vi "CheckChecksum.vi"(8 "error in (no error)":errorcluster, 11 "CS++Message in":refnum<class "CS++Message.lvclass">) -> (0 "error out":errorcluster, 2 "ok?":bool, 3 "CS++Message out":refnum<class "CS++Message.lvclass">)   [LabVIEW 2015, in "CS++Message.lvlib" / "CS++Message.lvclass"]
uses:
  CS++Message.lvclass
  CS++Message.lvclass/CS++Message.ctl
  <vilib>/Utility/traverseref.llb/TRef TravTarget.ctl
  <vilib>/Utility/traverseref.llb/VI Scripting - Traverse.lvlib
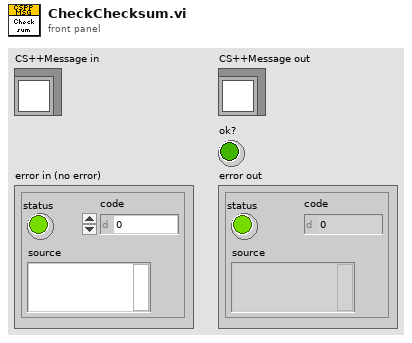
[diagram p1: front panel]
types:
  T1 = typedef "TRef TravTarget.ctl" = enum16{"FP", "BD", "Other"}
  T2 = typedef "imagedata.ctl" = cluster{"image type":i32, "image depth":i32, "image":u8[], "mask":u8[], "colors":u32[], "Rectangle":cluster{"left":i16, "top":i16, "right":i16, "bottom":i16}}
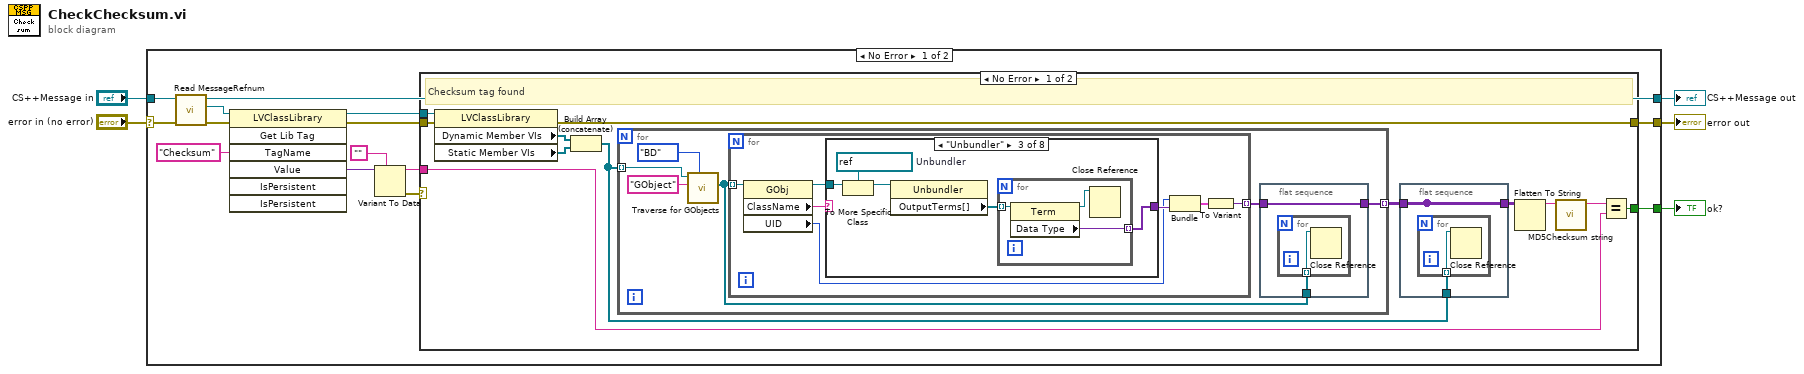
[diagram p0: block diagram]
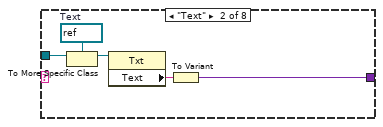
[diagram p3: hidden frame]
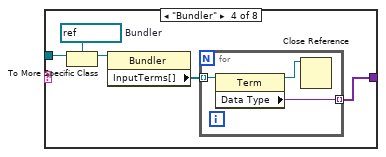
[diagram p4: hidden frame]
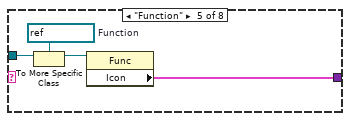
[diagram p5: hidden frame]
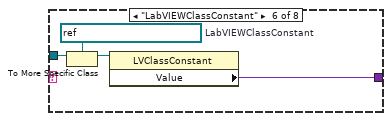
[diagram p6: hidden frame]
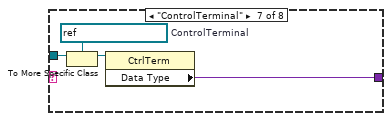
[diagram p7: hidden frame]
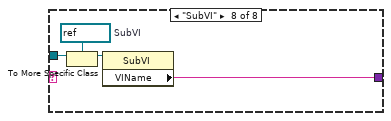
[diagram p8: hidden frame]
diagram:
  n1 = case shown="No Error" "error in (no error)" {
    selector: "error in (no error)" -> [w14 w90]
    tunnel: [w9 w90] -> w4
    tunnel: [w15 w89] -> w2
    tunnel: "CS++Message in" -> [w16 w89]
    tunnel: [w7 _] -> w1
    frame No Error {
      n2 = call "Read MessageRefnum.vi"("error in (no error)"=w14, "CS++Message in"=w16) -> ("error out"=w12:errorcluster, "MessageRefnum"=w13:refnum<vi>, "CS++Message out"=w15:refnum<class "CS++Message.lvclass">)  [unwired: 7 in]
      n3 = invoke class="LVClassLibrary" method="Get Lib Tag"(reference=w13, error in=w12, "TagName"="Checksum" ("Tag Name")) -> (reference out=w11:refnum<vi>, error out=w10:errorcluster, "Value"=w18:variant)  [unwired: 4 in, 4 out]
      n4 = Variant To Data(type="", Variant=w18) -> (data=w8:string, error out=w6:errorcluster)  [unwired: 1 in]
      n5 = case shown="No Error" w6 {
        tunnel: w11 -> [w31 _]
        tunnel: w10 -> [w30 w88]
        tunnel: [w29 w88] -> w9
        tunnel: w8 -> [w21 _]
        tunnel: [w20 _] -> w7
        frame No Error {
          # "Checksum tag found"
          n6 = property class="LVClassLibrary"(reference=w31, error in=w30) -> (error out=w29:errorcluster, "Dynamic Member VIs"=w28:refnum<vi>[], "Static Member VIs"=w27:refnum<vi>[])  [unwired: 1 out]
          n7 = Build Array (concatenate)(w28, w27) -> (w23:refnum<vi>[])
          n8 = for {
            tunnel: w23 -> [w38] mode=indexing
            tunnel: [w37] -> w25 mode=indexing
            n9 = call <vilib>:"Traverse for GObjects.vi"("Traverse Target"=TRef_TravTarget."BD", "Class Name"="GObject", "VI Refnum"=w38) -> ("References"=w35:refnum<vi>[])  [unwired: 5 in, 3 out]
            n10 = for {
              tunnel: w35 -> [w50] mode=indexing
              tunnel: [w44] -> w36 mode=indexing
              n11 = property class="GObj"(reference=w50) -> (reference out=w49:refnum<vi>, "ClassName"=w48:string, "UID"=w46:i32)  [unwired: 1 in, 1 out]
              n12 = case shown="\"Unbundler\"" w48 {
                tunnel: w49 -> [_ w54 w59 w67 w74 w78 w82 w86]
                tunnel: [_ w51 w56 w64 w72 w77 w80 w84] -> w47
                frame Default {
                }
                frame "Text" {
                  w55 = refnum<vi> refnum  # Text
                  n13 = To More Specific Class(target class=w55, reference=w54) -> (specific class reference=w53:refnum<vi>)  [unwired: 1 in, 1 out]
                  n14 = property class="Txt"(reference=w53) -> ("Text"=w52:string)  [unwired: 1 in, 2 out]
                  n15 = To Variant(anything=w52) -> (Variant=w51:variant)
                }
                frame "Unbundler" {
                  w60 = refnum<vi> refnum  # Unbundler
                  n16 = To More Specific Class(target class=w60, reference=w59) -> (specific class reference=w58:refnum<vi>)  [unwired: 1 in, 1 out]
                  n17 = property class="Unbundler"(reference=w58) -> ("OutputTerms[]"=w57:refnum<vi>[])  [unwired: 1 in, 2 out]
                  n18 = for {
                    tunnel: w57 -> [w63] mode=indexing
                    tunnel: [w62] -> w56 mode=indexing
                    n19 = property class="Term"(reference=w63) -> (reference out=w61:refnum<vi>, "Data Type"=w62:variant)  [unwired: 1 in, 1 out]
                    n20 = Close Reference(reference=w61) -> ()  [unwired: 1 in, 1 out]
                  }
                }
                frame "Bundler" {
                  w68 = refnum<vi> refnum  # Bundler
                  n21 = To More Specific Class(target class=w68, reference=w67) -> (specific class reference=w66:refnum<vi>)  [unwired: 1 in, 1 out]
                  n22 = property class="Bundler"(reference=w66) -> ("InputTerms[]"=w65:refnum<vi>[])  [unwired: 1 in, 2 out]
                  n23 = for {
                    tunnel: w65 -> [w71] mode=indexing
                    tunnel: [w70] -> w64 mode=indexing
                    n24 = property class="Term"(reference=w71) -> (reference out=w69:refnum<vi>, "Data Type"=w70:variant)  [unwired: 1 in, 1 out]
                    n25 = Close Reference(reference=w69) -> ()  [unwired: 1 in, 1 out]
                  }
                }
                frame "Function" {
                  w75 = refnum<vi> refnum  # Function
                  n26 = To More Specific Class(target class=w75, reference=w74) -> (specific class reference=w73:refnum<vi>)  [unwired: 1 in, 1 out]
                  n27 = property class="Func"(reference=w73) -> ("Icon"=w72:T2)  [unwired: 1 in, 2 out]
                }
                frame "LabVIEWClassConstant" {
                  w79 = refnum<vi> refnum  # LabVIEWClassConstant
                  n28 = To More Specific Class(target class=w79, reference=w78) -> (specific class reference=w76:refnum<vi>)  [unwired: 1 in, 1 out]
                  n29 = property class="LVClassConstant"(reference=w76) -> ("Value"=w77:variant)  [unwired: 1 in, 2 out]
                }
                frame "ControlTerminal" {
                  w83 = refnum<vi> refnum  # ControlTerminal
                  n30 = To More Specific Class(target class=w83, reference=w82) -> (specific class reference=w81:refnum<vi>)  [unwired: 1 in, 1 out]
                  n31 = property class="CtrlTerm"(reference=w81) -> ("Data Type"=w80:variant)  [unwired: 1 in, 2 out]
                }
                frame "SubVI" {
                  w87 = refnum<vi> refnum  # SubVI
                  n32 = To More Specific Class(target class=w87, reference=w86) -> (specific class reference=w85:refnum<vi>)  [unwired: 1 in, 1 out]
                  n33 = property class="SubVI"(reference=w85) -> ("VIName"=w84:string)  [unwired: 1 in, 2 out]
                }
              }
              n34 = Bundle("UID"=w46, "Data Type"=w47) -> (w45:cluster{"UID":i32, "Data Type":variant})  [unwired: 1 in]
              n35 = To Variant(anything=w45) -> (Variant=w44:variant)
            }
            n36 = flat-sequence {
              tunnel: [w42] -> w37
              tunnel: w36 -> [w42]
              tunnel: w35 -> [w41]
              frame #0 {
                n37 = for {
                  tunnel: w41 -> [w43] mode=indexing
                  n38 = Close Reference(reference=w43) -> ()  [unwired: 1 in, 1 out]
                }
              }
            }
          }
          n39 = flat-sequence {
            tunnel: [w32] -> _
            tunnel: w25 -> [w32]
            tunnel: w23 -> [w33]
            tunnel: [w32] -> w24
            frame #0 {
              n40 = for {
                tunnel: w33 -> [w34] mode=indexing
                n41 = Close Reference(reference=w34) -> ()  [unwired: 1 in, 1 out]
              }
            }
          }
          n42 = Flatten To String(anything=w24) -> (data string=w26:string)  [unwired: 3 in, 2 out]
          n43 = call <vilib>:"MD5Checksum string.vi"("Message String"=w26) -> ("MD5 message-digest"=w22:string)  [unwired: 10 in]
          n44 = Equal?(x=w22, y=w21) -> (x = y?=w20:bool)
        }
        frame Error {
          # "Checksum tag not found"
        }
      }
    }
    frame Error {
    }
  }
  "error out" <- w4
  "CS++Message out" <- w2
  "ok?" <- w1
